vi "Simulator PIM Unflatten Driver Configuration.vi"(9 "PIM Configuration (\"\")":string) -> (1 "Configuration":T1={"host IP (localhost)"="localhost", "host Port"=3388, "Model"="", "Serial Number(s)"="", "Calibration Date"=3388.0, "Dual Port?"=FALSE, "DeviceNames"=[], "Parameters"={"TX1start"=0.0, "TX1stop"=0.0, "TX1pmax"=0.0, "TX2start"=0.0, "TX2stop"=0.0, "TX2pmax"=0.0, "RXstart"=0.0, "RXstop"=0.0}, "Interface"=enum."PIM Web Engine"} {"Calibration Date" format="%.2f"; "Parameters"."TX2pmax" format="%.1f"; "Parameters"."TX1pmax" format="%.1f"; "Parameters"."RXstop" format="%.1f"; "Parameters"."RXstart" format="%.1f"; "Parameters"."TX2stop" format="%.1f"; "Parameters"."TX2start" format="%.1f"; "Parameters"."TX1stop" format="%.1f"; "Parameters"."TX1start" format="%.1f"}, 4 "Version":string)   [LabVIEW 2011]
uses:
  PIM Configuration.ctl
  PIM Interface Language.ctl
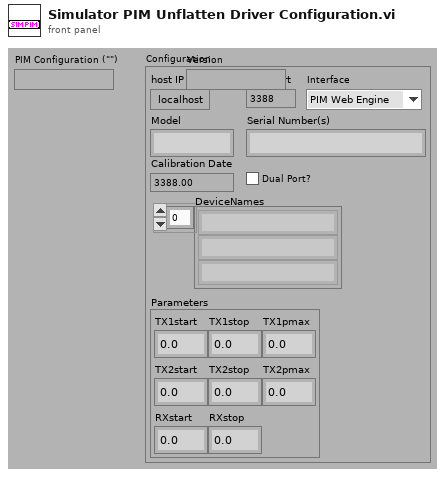
[diagram p1: front panel]
types:
  T1 = typedef "PIM Configuration.ctl" = cluster{"host IP (localhost)":string, "host Port":u16, "Model":string, "Serial Number(s)":string, "Calibration Date":dbl, "Dual Port?":bool, "DeviceNames":string[], "Parameters":cluster{"TX1start":dbl, "TX1stop":dbl, "TX1pmax":dbl, "TX2start":dbl, "TX2stop":dbl, "TX2pmax":dbl, "RXstart":dbl, "RXstop":dbl}, "Interface":T2}
  T2 = typedef "PIM Interface Language.ctl" = enum16{"PIM Web Engine", "PIM HW Engine"}
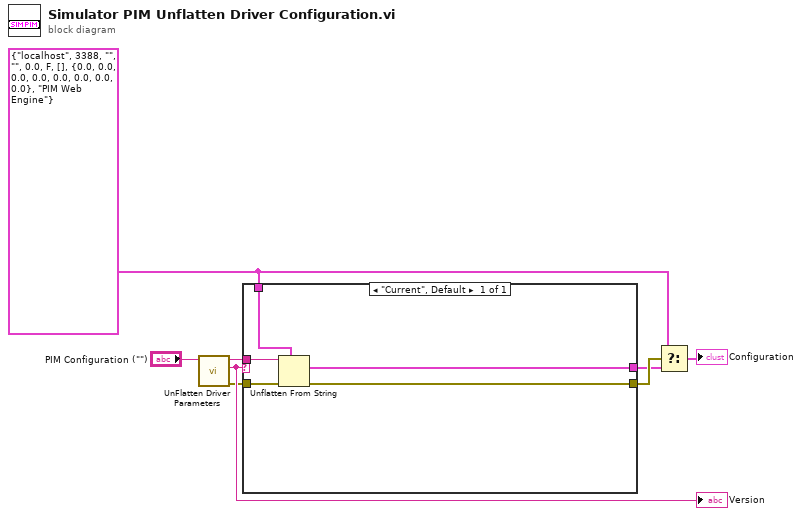
[diagram p0: block diagram]
diagram:
  w1 = T1 {"host IP (localhost)"="localhost", "host Port"=3388, "Model"="", "Serial Number(s)"="", "Calibration Date"=0.0, "Dual Port?"=FALSE, "DeviceNames"=[], "Parameters"={"TX1start"=0.0, "TX1stop"=0.0, "TX1pmax"=0.0, "TX2start"=0.0, "TX2stop"=0.0, "TX2pmax"=0.0, "RXstart"=0.0, "RXstop"=0.0}, "Interface"=enum."PIM Web Engine"} ("PIM Configuration")
  n1 = call "UnFlatten Driver Parameters.vi"("Flattened Driver Parameters with Version (\"\")"="PIM Configuration (\"\")") -> ("error out"=w3:errorcluster, "Driver Version"=w8:string, "Flat Driver Parameters"=w7:string)  [unwired: 1 in, 3 out]
  "Version" <- w8
  n2 = case shown="\"Current\", Default" w8 {
    tunnel: w7 -> [w13]
    tunnel: w1 -> [w12]
    tunnel: [w11] -> w5
    tunnel: [w10] -> w6
    tunnel: w3 -> [w9]
    frame "Current", Default {
      n3 = Unflatten From String(type=w12, binary string=w13, error in (no error)=w9) -> (value=w11:T1, error out=w10:errorcluster)  [unwired: 3 out]
    }
  }
  n4 = Select(t=w1, s=w6, f=w5) -> (s? t:f=→"Configuration":T1)
